vi "PriceData Randomize Energy.vi"(10 "DeviceID":T2) -> (3 "PriceData_Energy Array out":T1[](array[typedef]))   [LabVIEW 2018, in "IED Test Framework.lvlib" / "IED Test.lvclass"]
uses:
  IED Test.lvclass
  <vilib>/ORNL/CSEISMIC DDS/CSEISMIC DDS Base/Data Types/Controls/DeviceID.ctl
  <vilib>/ORNL/CSEISMIC DDS/CSEISMIC DDS Base/Data Types/PriceData_Energy.ctl
  <vilib>/ORNL/CSEISMIC DDS/CSEISMIC DDS Base/CSEISMIC DDS.lvclass
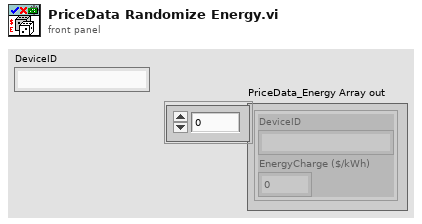
[diagram p1: front panel]
types:
  T1 = typedef "CSEISMIC DDS.lvlib/CSEISMIC DDS.lvclass/PriceData_Energy.ctl" = cluster{"DeviceID":T2, "EnergyCharge ($/kWh)":dbl}
  T2 = typedef "CSEISMIC DDS.lvlib/CSEISMIC DDS.lvclass/DeviceID.ctl" = string
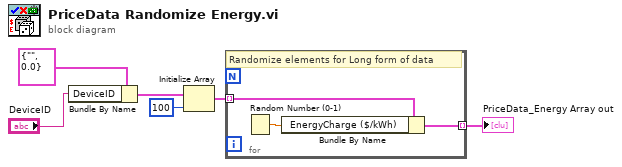
[diagram p0: block diagram]
diagram:
  n1 = Bundle By Name(cluster=T1 {"DeviceID"="", "EnergyCharge ($/kWh)"=0.0} ("PriceData_Energy"), "DeviceID"="DeviceID") -> (w6:T1)
  n2 = Initialize Array(w6, 100 ("dimension size")) -> (w3:T1[])
  n3 = for {
    tunnel: w3 -> [w9] mode=indexing
    tunnel: [w8] -> w2 mode=indexing
    # "Randomize elements for Long form of data"
    n4 = Random Number (0-1)() -> (number: 0 to 1=w7:dbl)
    n5 = Bundle By Name(cluster=w9, "EnergyCharge ($/kWh)"=w7) -> (w8:T1)
  }
  "PriceData_Energy Array out" <- w2
